vi "set value.vi"(8 "error in":errorcluster, 9 "value":variant, 10 "value index":i32, 11 "displayable in":refnum<class "displayable.lvclass">) -> (0 "error out":errorcluster, 3 "displayable out":refnum<class "displayable.lvclass">)   [LabVIEW 2013, in "displayable.lvclass"]
uses:
  displayable.lvclass
  displayable.lvclass/displayable.ctl
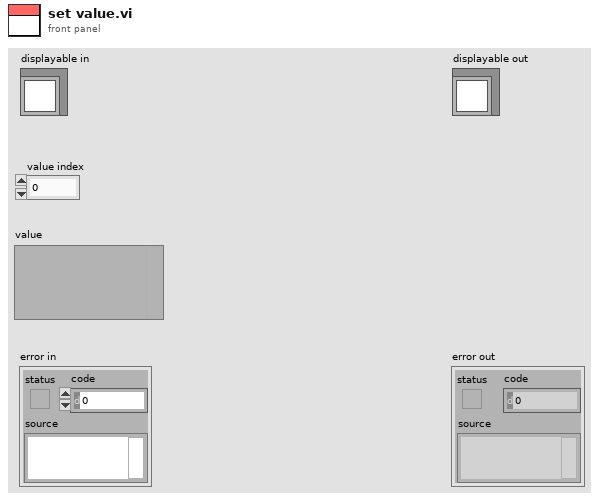
[diagram p1: front panel]
types:
  T1 = typedef "displayable.lvclass/subscription.ctl" = cluster{"control indexes":i32[]}
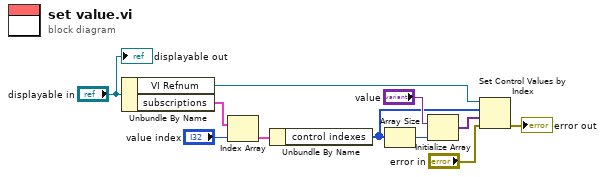
[diagram p0: block diagram]
diagram:
  n1 = Unbundle By Name("displayable in") -> ("VI Refnum"=w3:refnum<vi>, "subscriptions"=w10:T1[])
  n2 = Index Array(array=w10, index="value index") -> (element=w8:T1)
  n3 = Unbundle By Name(w8) -> ("control indexes"=w4:i32[])
  n4 = Array Size(array=w4) -> (size(s)=w7:i32)
  n5 = Initialize Array("value", w7) -> (w5:variant[])
  n6 = Set Control Values by Index(0:w3, 1:w4, 2:w5, 3:"error in") -> (11:→"error out":errorcluster)
  "displayable out" <- "displayable in"
